vi "main.vi"() -> ()   [LabVIEW 2019]
panel:
  in  "Krok [mA]":u32
  in  "Wartoœæ  koñcowa [mA]":u32
  out "Info":string
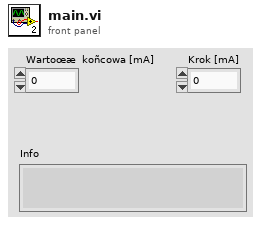
[diagram p1: front panel]
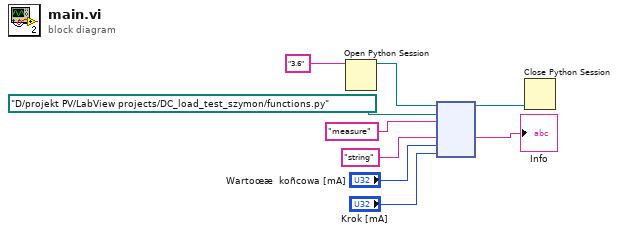
[diagram p0: block diagram]
diagram:
  n1 = Open Python Session(python version="3.6" ("Python version")) -> (session out=w6:refnum<k35>)  [unwired: 2 in, 1 out]
  n2 = node(w6, path "D:/projekt PV/LabView projects/DC_load_test_szymon/functions.py" ("module path"), "measure" ("function name"), "string" ("function name"), "Wartoœæ  koñcowa [mA]", "Krok [mA]") -> (w5:refnum<k35>, →"Info":string)  [unwired: 3 in, 3 out]
  n3 = Close Python Session(session in=w5) -> ()  [unwired: 1 in, 1 out]
